vi "PE7260_setup.vi"(2 "PE7625-Settings":T1={"PE7265 AutoSens at ech step"=FALSE, "PE7265 Sens"=26, "Coupling"=FALSE, "AC Gain"=3, "Auto AC Gain"=FALSE, "Input Device (Voltage Mode)"=TRUE, "Line Frequency"=TRUE, "Input Connector Shells"=FALSE, "PE7265 Input Mode"=3, "Line Frequency\nRejection Filter"=1, "Port"=0, "7265 GPIB Address"=12, "Interface"=FALSE, "Exit"=FALSE, "GPIB Parameter 7260"={"address"="12", "delay time"=10.0, "mode"=6}, "PE7265 delay after AS"=10.0, "VISA session PE7265"="GPIB0::12::INSTR", "Slope"=1, "Synchronous TC"=TRUE, "Time Constant"=15, "Reference I/P"=0, "Reference\nHarmonic"=1, "Oscillator Amplitude (Volts rms)"=1.5, "Oscillator Frequency (Hz)"=19.0, "Ref Unlocked"=FALSE, "Virtual Reference\nMode"=FALSE} {"Oscillator Frequency (Hz)" min=0.001 max=250000.0 step=0.001 format="%.3f"; "Oscillator Amplitude (Volts rms)" min=0.0 max=5.0 step=1e-06 format="%.6f"; "Reference\nHarmonic" min=1 step=1; "Reference I/P" items=["Internal", "External TTL (Rear Panel)", "External (Front Panel)"]; "Time Constant" items=["10µs", "20µs", "40µs", "80µs", "160µs", "320µs", "640µs", "5ms", "10ms", "20ms", "50ms", "100ms", "200ms", "500ms", "1s", "2s", "5s", "10s", "20s", "50s", "100s", "200s", "500s", "1ks", "2ks", "5ks", "10ks", "20ks", "50ks", "100ks"]; "Slope" items=["6db/octave", "12dB/octave", "18dB/octave", "24dB/octave"]; "PE7265 delay after AS" format="%.2f"; "GPIB Parameter 7260"."delay time" format="%.2f"; "7265 GPIB Address" min=1 max=32 step=1; "Port" items=["COM 1", "COM 2", "COM 3", "COM 4", "COM 5", "COM 6", "COM 7", "COM 8", "COM 9", "COM 10"]; "Line Frequency\nRejection Filter" items=["OFF", "F", "2F", "F & 2F"]; "PE7265 Input Mode" items=["Inputs Grounded (test)", "A (Single-Ended Voltage)", "-B (Inverting Single Ended Voltage)", "A-B (Differential Voltage)", "B Current input - High Bandwidth", "B Current input - Low Noise"]; "AC Gain" items=["0dB", "10dB", "20dB", "30dB", "40dB", "50dB", "60dB", "70dB", "80dB", "90dB"]; "PE7265 Sens" items=["2nV", "5nV", "10nV", "20nV", "50nV", "100nV", "200nV", "500nV", "1µV", "2µV", "5µV", "10µV", "20µV", "50µV", "100µV", "200µV", "500µV", "1mV", "2mV", "5mV", "10mV", "20mV", "50mV", "100mV", "200mV", "500mV", "1V"]}) -> ()   [LabVIEW 2018]
uses:
  PE7625-Settings.ctl
panel:
  # "Input Configuration"
  # "RS232"
  # "GPIB"
  # "Uses VISA Communications"
  # "Sensitivity"
  # "Float"
  # "50 Hz"
  # "DC"
  # "Ground"
  # "60 Hz"
  # "AC"
  # "Bipolar - Input Impedance 10 k"
  # "On"
  # "FET - Input Impedance 10 M"
  # "Off"
  # "Output Channels"
  # "Reference Channel - Single Reference"
  # "On"
  # "Off"
  # "On"
  # "Off"
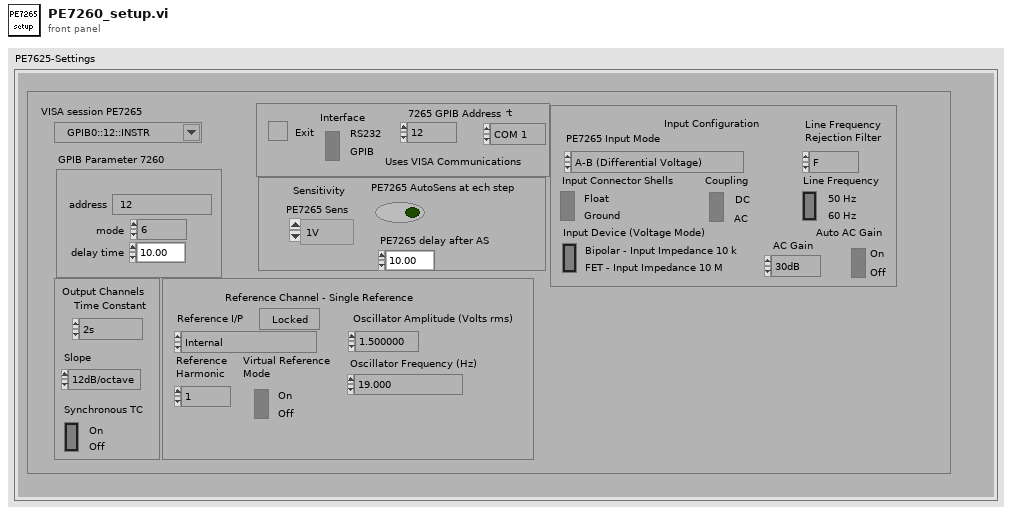
[diagram p1: front panel]
types:
  T1 = typedef "PE7625-Settings.ctl" = cluster{"PE7265 AutoSens at ech step":bool, "PE7265 Sens":i32, "Coupling":bool, "AC Gain":u16, "Auto AC Gain":bool, "Input Device (Voltage Mode)":bool, "Line Frequency":bool, "Input Connector Shells":bool, "PE7265 Input Mode":u16, "Line Frequency\nRejection Filter":u8, "Port":u16, "7265 GPIB Address":i8, "Interface":bool, "Exit":bool, "GPIB Parameter 7260":cluster{"address":string, "delay time":dbl, "mode":i32}, "PE7265 delay after AS":dbl, "VISA session PE7265":refnum<visa-resource-name>, "Slope":u8, "Synchronous TC":bool, "Time Constant":u16, "Reference I/P":u8, "Reference\nHarmonic":u16, "Oscillator Amplitude (Volts rms)":dbl, "Oscillator Frequency (Hz)":dbl, "Ref Unlocked":bool, "Virtual Reference\nMode":bool}
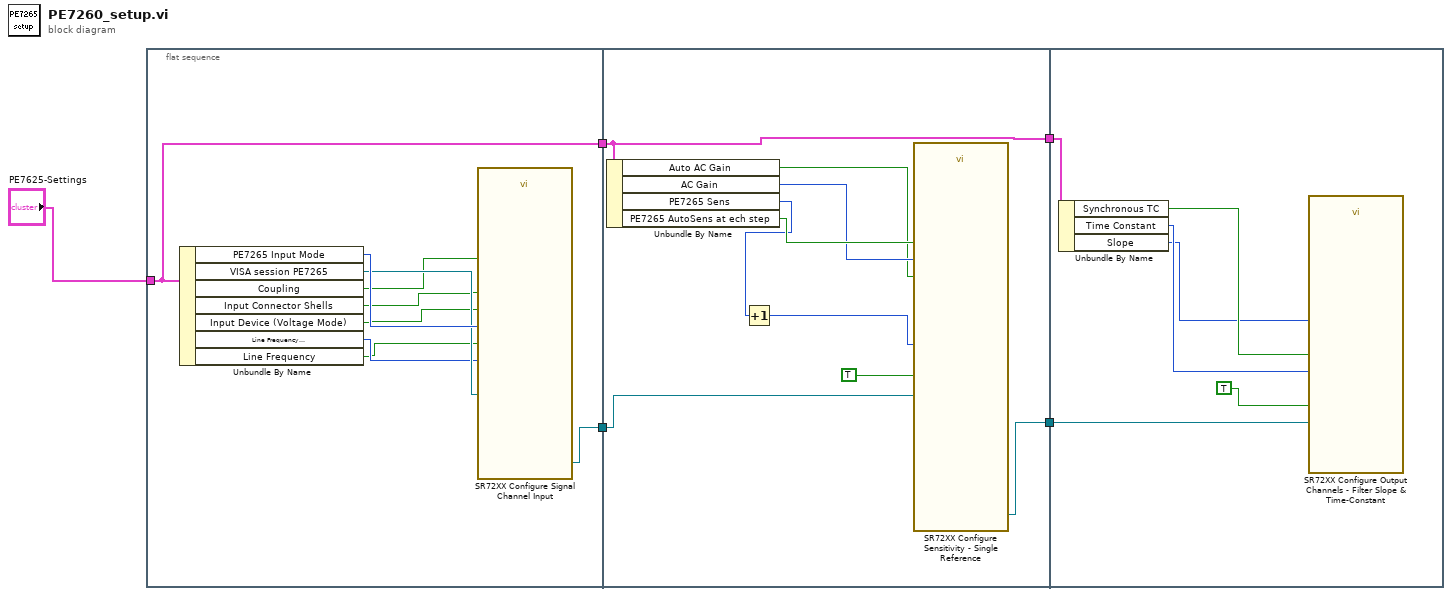
[diagram p0: block diagram]
diagram:
  n1 = flat-sequence {
    tunnel: "PE7625-Settings" -> [w7]
    tunnel: [w7] -> w4
    tunnel: [w6] -> w3
    tunnel: w4 -> [w15]
    tunnel: w3 -> [w23]
    tunnel: [w16] -> w2
    tunnel: [w15] -> w1
    tunnel: w2 -> [w29]
    tunnel: w1 -> [w27]
    frame #0 {
      n2 = Unbundle By Name(w7) -> ("PE7265 Input Mode"=w14:u16, "VISA session PE7265"=w13:refnum<visa-resource-name>, "Coupling"=w12:bool, "Input Connector Shells"=w11:bool, "Input Device (Voltage Mode)"=w10:bool, "Line Frequency\nRejection Filter"=w9:u8, "Line Frequency"=w8:bool)
      n3 = call "SR72XX Configure Signal Channel Input.vi"("VISA session (for class)"=w13, "Input Mode"=w14, "Input Connector Shells"=w11, "Input Device (Voltage Mode)"=w10, "Line Frequency"=w8, "Line Frequency Rejection Filter"=w9, "Coupling"=w12) -> ("VISA session"=w6:refnum<visa-resource-name>)  [unwired: 9 in, 3 out]
    }
    frame #1 {
      n4 = Unbundle By Name(w15) -> ("Auto AC Gain"=w20:bool, "AC Gain"=w21:u16, "PE7265 Sens"=w19:i32, "PE7265 AutoSens at ech step"=w22:bool)
      n5 = Increment(x=w19) -> (x+1=w18:i32)
      n6 = call "SR72XX Configure Sensitivity - Single Reference.vi"("VISA session (for class)"=w23, "AC Gain"=w21, "Auto AC Gain"=w20, "Range"=w18, "Auto Sensitivity"=w22, "Update"=TRUE) -> ("VISA session"=w16:refnum<visa-resource-name>)  [unwired: 7 in, 6 out]
    }
    frame #2 {
      n7 = Unbundle By Name(w27) -> ("Synchronous TC"=w26:bool, "Time Constant"=w25:u16, "Slope"=w24:u8)
      n8 = call "SR72XX Configure Output Channels - Filter Slope & Time-Constant.vi"("VISA session (for class)"=w29, "Time Constant"=w25, "Slope"=w24, "Synchronous TC"=w26, "Update"=TRUE) -> ()  [unwired: 13 in, 2 out]
    }
  }
